vi "Set_FlyWheelOutput.vi"(11 "FlyWheelOutputs":T1) -> (0 "error out":errorcluster)   [LabVIEW 2012]
uses:
  Outputs_Flywheel.ctl
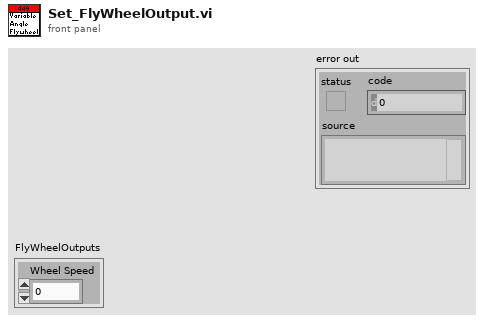
[diagram p1: front panel]
types:
  T1 = typedef "Outputs_Flywheel.ctl" = cluster{"Wheel Speed":dbl}
  T2 = typedef "WPI_MotorControlDeviceRef.ctl" = cluster{"DeviceStatus":errorcluster, "Type":enum16{"PWM", "CAN"}, "PWM":cluster{"Digital Module":T3, "PWM Channel":T4, "DeadBand":T5}, "CAN":cluster{"Device Number":u8, "Control Mode":T6, "Semaphore":T7, "Max Vout":dbl}, "Invert":bool, "TransformRef":T8, "InvTransformRef":T8}
  T3 = typedef "FPGA_TypedefDigitalModule.ctl" = enum16{"Digital Module 1", "Digital Module 2"}
  T4 = typedef "FPGA_DIOPWMChannel.ctl" = enum8{"PWM 1", "PWM 2", "PWM 3", "PWM 4", "PWM 5", "PWM 6", "PWM 7", "PWM 8", "PWM 9", "PWM 10", "Invalid"}
  T5 = typedef "WPI_PWMDeadband.ctl" = cluster{"Name":string, "maxPositivePwm":i32, "minPositivePwm":i32, "centerPwm":i32, "maxNegativePwm":i32, "minNegativePwm":i32, "angularRange":u16}
  T6 = typedef "WPI_CANJaguar_ControlMode.ctl" = enum8{"Percent VBus", "Current", "Speed", "Position", "Voltage"}
  T7 = typedef "Semaphore RefNum" = refnum<k1>
  T8 = typedef "WPI_PWMTransform_ConPane.ctl" = refnum<vi>
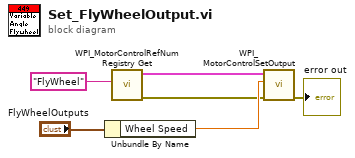
[diagram p0: block diagram]
diagram:
  n1 = Unbundle By Name("FlyWheelOutputs") -> ("Wheel Speed"=w3:dbl)
  n2 = call <vilib>:"WPI_MotorControlRefNum Registry Get.vi"("refnum name"="FlyWheel") -> ("error out"=w2:errorcluster, "MotorControlDevRef"=w5:T2)  [unwired: 9 in]
  n3 = call <vilib>:"WPI_MotorControlSetOutput.vi"("error in (no error)"=w2, "Output"=w3, "MotorControlDevRef"=w5) -> ("error out"=→"error out":errorcluster)  [unwired: 6 in, 2 out]
